vi "HXG2_PassSetPoints.vi"(7 "Run Programmer":bool, 8 "error in (no error)":errorcluster, 9 "Air Cluster Ref":refnum<vi>, 10 "Gly Cluster Ref":refnum<vi>, 11 "AIR-GLY Cluster In":T2 {"Liq Cluster"."Liq TEMP %" min=0.0 max=100.0 step=1.0 format="%#.1f"; "Liq Cluster"."Liq FLOW %" min=0.0 max=100.0 step=1.0 format="%#.1f"; "Liq Cluster"."TLiq °F" min=40.0 max=180.0 step=1.0 format="%#.1f"; "Liq Cluster"."Mdot lbm/hr" min=0.0 max=1000.0 step=1.0 format="%#.1f"; "Air Cluster"."Air TEMP %" min=0.0 max=100.0 step=1.0 format="%#.1f"; "Air Cluster"."Air FLOW %" min=0.0 max=100.0 step=1.0 format="%#.1f"; "Air Cluster"."Tair  °F" min=-5.0 max=100.0 step=1.0 format="%#.1f"; "Air Cluster"."CFMs" min=0.0 max=200.0 step=1.0 format="%#.1f"}) -> (0 "error out":errorcluster, 2 "Setpoints":T1, 3 "AIR-GLY Cluster Out":T2 {"Liq Cluster"."Liq TEMP %" min=0.0 max=100.0 step=1.0 format="%#.1f"; "Liq Cluster"."Liq FLOW %" min=0.0 max=100.0 step=1.0 format="%#.1f"; "Liq Cluster"."TLiq °F" min=40.0 max=180.0 step=1.0 format="%#.1f"; "Liq Cluster"."Mdot lbm/hr" min=0.0 max=1000.0 step=1.0 format="%#.1f"; "Air Cluster"."Air TEMP %" min=0.0 max=100.0 step=1.0 format="%#.1f"; "Air Cluster"."Air FLOW %" min=0.0 max=100.0 step=1.0 format="%#.1f"; "Air Cluster"."Tair  °F" min=-5.0 max=100.0 step=1.0 format="%#.1f"; "Air Cluster"."CFMs" min=0.0 max=200.0 step=1.0 format="%#.1f"})   [LabVIEW 2012]
doc: "Passes setpoints based on programmer table\nRuns the Programmer FGV in Execute Programmer state"
uses:
  Controls/HXG2_AirGly-Cluster.ctl
  Controls/UI/HXG2_UI_ControlSetAir.ctl
  Controls/UI/HXG2_UI_ControlSetGly.ctl
  Modules/Programmer/Data Types/Programmer Execution States.ctl
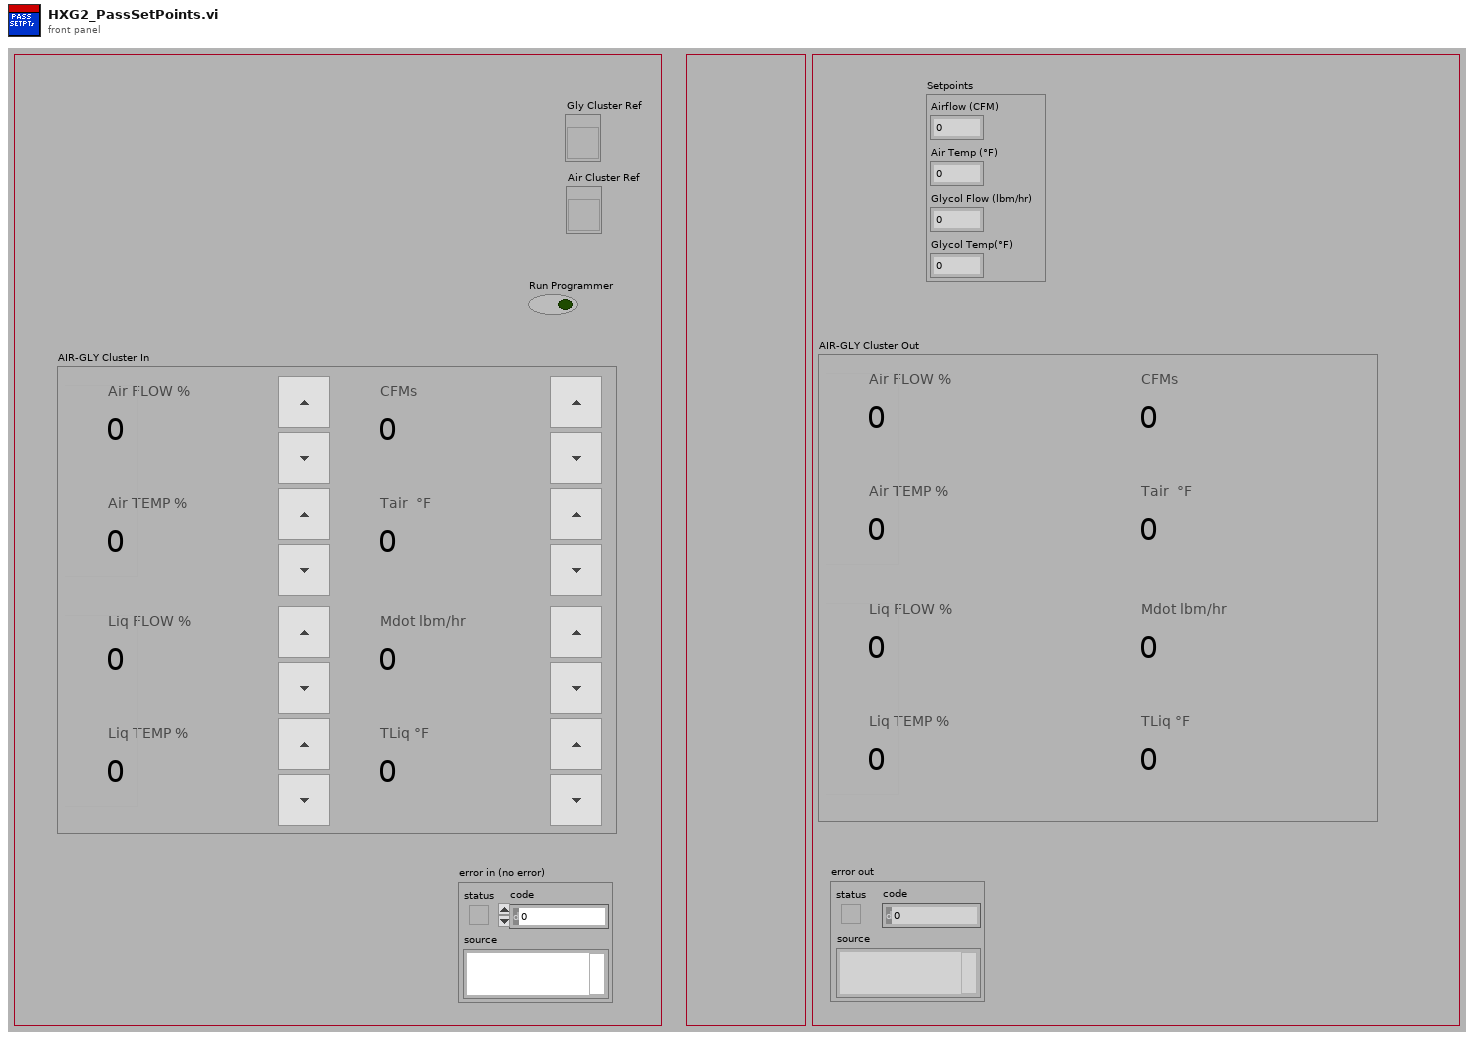
[diagram p1: front panel]
types:
  T1 = cluster{"Airflow (CFM)":dbl, "Air Temp (°F)":dbl, "Glycol Flow (lbm/hr)":dbl, "Glycol Temp(°F)":dbl}
  T2 = typedef "HXG2_AirGly-Cluster.ctl" = cluster{"Air Cluster":T3, "Liq Cluster":T4}
  T3 = typedef "HXG2_UI_ControlSetAir.ctl" = cluster{"Air FLOW %":dbl, "Air TEMP % ":dbl, "CFMs":dbl, "Tair  °F":dbl}
  T4 = typedef "HXG2_UI_ControlSetGly.ctl" = cluster{"Liq FLOW %":dbl, "Liq TEMP % ":dbl, "Mdot lbm/hr":dbl, "TLiq °F":dbl}
  T5 = typedef "Programmer Execution States.ctl" = enum16{"Register Steps", "Initialize", "Start Test Sequence", "Register Data", "Execute Programmer", "Set Number of Repetitions", "Get Current Step Index", "Get Time Until Step Ends"}
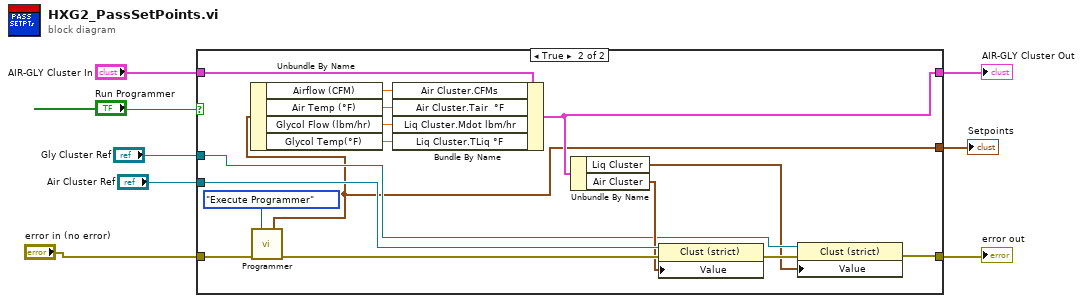
[diagram p0: block diagram]
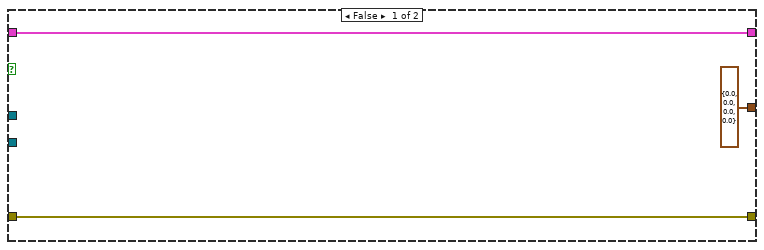
[diagram p2: hidden frame]
diagram:
  n1 = case shown="True" "Run Programmer" {
    tunnel: "AIR-GLY Cluster In" -> [w11 w27]
    tunnel: [w11 w18] -> w7
    tunnel: "error in (no error)" -> [w10 w22]
    tunnel: [w10 w15] -> w4
    tunnel: "Air Cluster Ref" -> [_ w19]
    tunnel: "Gly Cluster Ref" -> [_ w14]
    tunnel: [T1 {"Airflow (CFM)"=0.0, "Air Temp (°F)"=0.0, "Glycol Flow (lbm/hr)"=0.0, "Glycol Temp(°F)"=0.0} ("Setpoints") w12] -> w1
    frame False {
    }
    frame True {
      n2 = call "Programmer.vi"("Action"=Programmer_Execution_States."Execute Programmer", "error in (no error)"=w22) -> ("Setpoints"=w12:T1, "error out"=w20:errorcluster)  [unwired: 6 in, 6 out]
      n3 = Unbundle By Name(w12) -> ("Airflow (CFM)"=w26:dbl, "Air Temp (°F)"=w25:dbl, "Glycol Flow (lbm/hr)"=w24:dbl, "Glycol Temp(°F)"=w23:dbl)
      n4 = Bundle By Name(cluster=w27, "Air Cluster.CFMs"=w26, "Air Cluster.Tair  °F"=w25, "Liq Cluster.Mdot lbm/hr"=w24, "Liq Cluster.TLiq °F"=w23) -> (w18:T2)
      n5 = Unbundle By Name(w18) -> ("Liq Cluster"=w13:T4, "Air Cluster"=w17:T3)
      n6 = property class="Clust (strict)"(reference=w19, error in=w20, "Value"=w17) -> (error out=w16:errorcluster)  [unwired: 1 out]
      n7 = property class="Clust (strict)"(reference=w14, error in=w16, "Value"=w13) -> (error out=w15:errorcluster)  [unwired: 1 out]
    }
  }
  "AIR-GLY Cluster Out" <- w7
  "error out" <- w4
  "Setpoints" <- w1
